vi "RS232SerialPortTest.vi"   [LabVIEW 2016]
uses:
  Common_FPGA_Serial/DataTypes/SerialSettings.ctl
  Common_FPGA_Timestamp/DataTypes/TimestampSettings.ctl
  Common_FPGA_Serial/FPGASerial.lvlib
  Common_FPGA_Timestamp/FPGATimestamp.lvlib
types:
  T1 = typedef "FPGATimestamp.lvlib/TimestampSettings.ctl" = cluster{"TimeRegister":refnum<k21>, "TimeSource":refnum<k21>, "IterationsPerMicrosecond":i16, "UpdateFIFO":refnum<k21>}
  T2 = typedef "FPGASerial.lvlib/SerialSettings.ctl" = cluster{"SerialPort":refnum<k21>, "TxFIFO":refnum<k21>, "RxFIFO":refnum<k21>, "TimestampRegister":refnum<k21>}
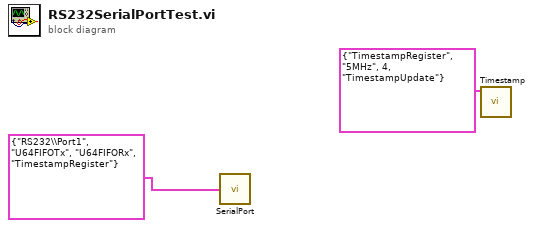
[diagram p0: block diagram]
diagram:
  n1 = call "SerialPort.vi"("SerialSettings"=T2 {"SerialPort"="RS232\\Port1", "TxFIFO"="U64FIFOTx", "RxFIFO"="U64FIFORx", "TimestampRegister"="TimestampRegister"}) -> ()  [unwired: 1 in]
  n2 = call "Timestamp.vi"("TimestampSettings"=T1 {"TimeRegister"="TimestampRegister", "TimeSource"="5MHz", "IterationsPerMicrosecond"=4, "UpdateFIFO"="TimestampUpdate"}) -> ()  [unwired: 11 in]
